vi "BallOutOfFieldRole.vi"(8 "error in (no error)":errorcluster, 10 "Game in":refnum<class "Game.lvclass">, 11 "BallOutOfFieldRole in":refnum<class "BallOutOfFieldRole.lvclass">) -> (0 "error out":errorcluster, 1 "Game out":refnum<class "Game.lvclass">, 2 "Robot out":refnum<class "Robot.lvclass">, 3 "BallOutOfFieldRole out":refnum<class "BallOutOfFieldRole.lvclass">)   [LabVIEW 2018, in "BallOutOfFieldRole.lvclass"]
uses:
  BallOutOfFieldRole.lvclass
  AttackerBallOutOfFieldTactic_class/AttackerBallOutOfFieldTactic.lvclass
  Tacticbook_class/Tacticbook.lvclass
  AttackerBallOutOfFieldTactic_class/States.ctl
  Game_class/Game.lvclass
  Robot_class/Robot.lvclass
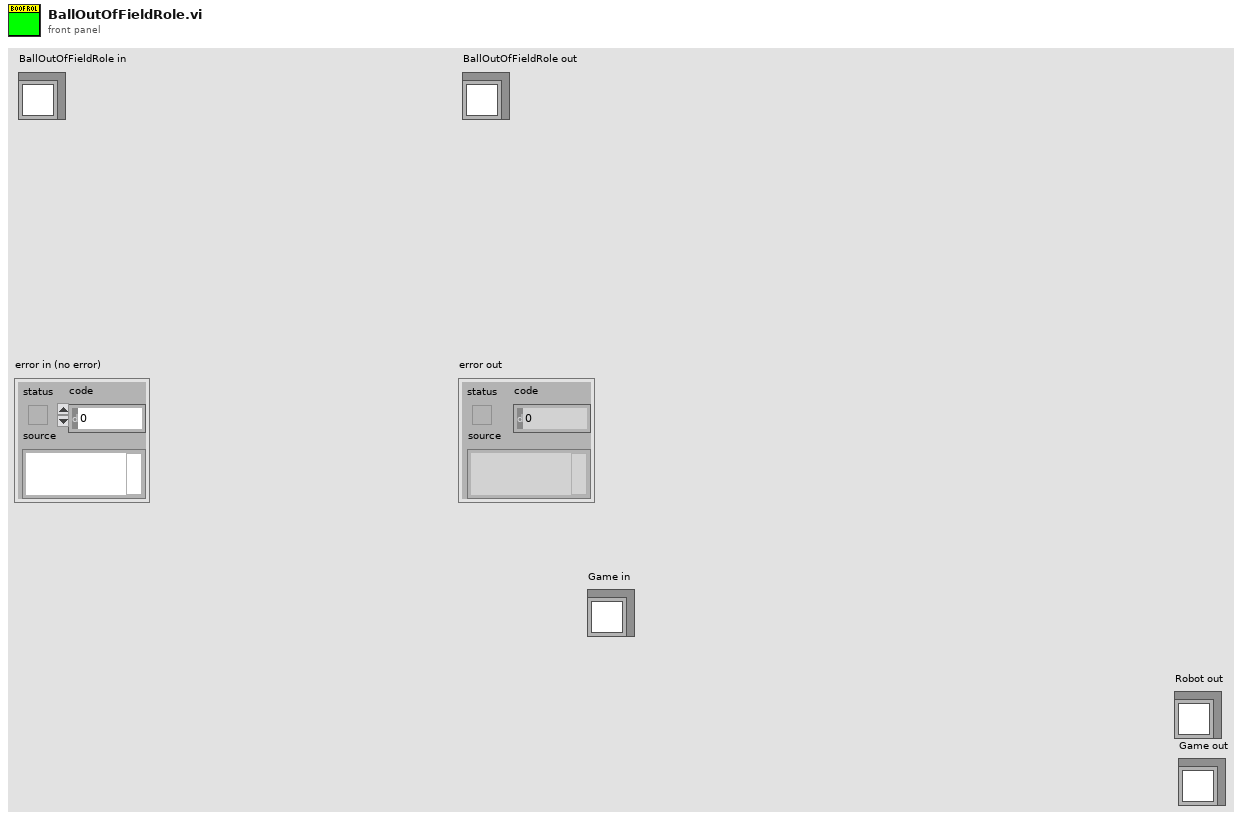
[diagram p1: front panel]
types:
  T1 = typedef "AttackerBallOutOfFieldTactic.lvclass/States.ctl" = enum16{"Exit", "BallOutOfField"}
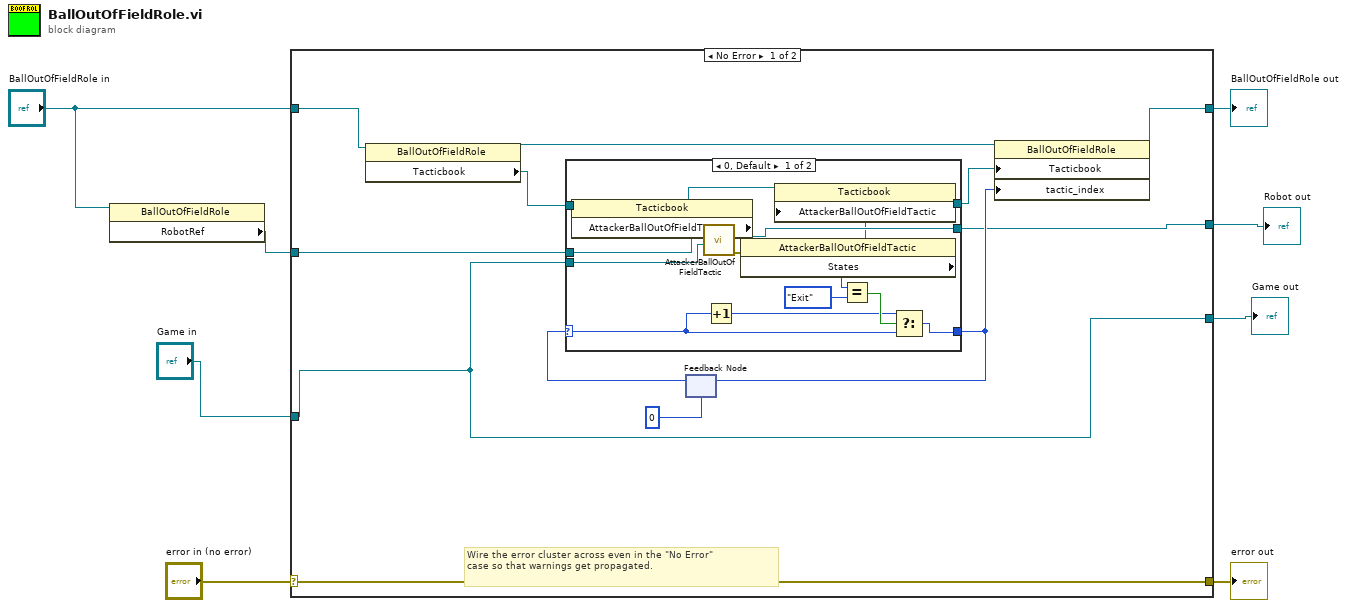
[diagram p0: block diagram]
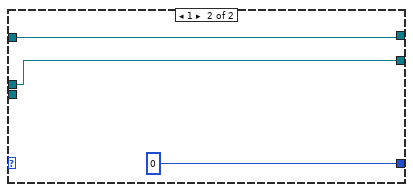
[diagram p2: hidden frame]
diagram:
  n1 = property class="BallOutOfFieldRole"(reference="BallOutOfFieldRole in") -> ("RobotRef"=w5:refnum<class "Robot.lvclass">)  [unwired: 1 in, 2 out]
  n2 = case shown="No Error" "error in (no error)" {
    selector: "error in (no error)" -> [w20 w43]
    tunnel: [w20 w43] -> w7
    tunnel: [w9 w42] -> w6
    tunnel: "BallOutOfFieldRole in" -> [w13 w42]
    tunnel: w5 -> [w12 w41]
    tunnel: "Game in" -> [w11 w40]
    tunnel: [w11 w40] -> w3
    tunnel: [w10 w41] -> w2
    frame No Error {
      # "Wire the error cluster across even in the \"No Error\"\ncase so that warnings get propagated."
      n3 = property class="BallOutOfFieldRole"(reference=w13) -> (reference out=w19:refnum<class "BallOutOfFieldRole.lvclass">, "Tacticbook"=w16:refnum<class "Tacticbook.lvclass">)  [unwired: 1 in, 1 out]
      n4 = feedback #1(0) -> (w17:i32)
      n5 = case shown="0, Default" w17 {
        selector: w17 -> [w27 _]
        tunnel: [w28 0] -> w15
        tunnel: w16 -> [w36 w37]
        tunnel: w12 -> [w34 w39]
        tunnel: [w33 w39] -> w10
        tunnel: [w23 w37] -> w14
        tunnel: w11 -> [w22 _]
        frame 0, Default {
          n6 = property class="Tacticbook"(reference=w36) -> (reference out=w25:refnum<class "Tacticbook.lvclass">, "AttackerBallOutOfFieldTactic"=w35:refnum<class "AttackerBallOutOfFieldTactic.lvclass">)  [unwired: 1 in, 1 out]
          n7 = call-dynamic "AttackerBallOutOfFieldTactic.vi"("Game in"=w22, "Robot"=w34, "AttackerBallOutOfFieldTactic in"=w35) -> ("error out"=w32:errorcluster, "Robot out"=w33:refnum<class "Robot.lvclass">, "AttackerBallOutOfFieldTactic out"=w31:refnum<class "AttackerBallOutOfFieldTactic.lvclass">)  [unwired: 6 in]
          n8 = Increment(x=w27) -> (x+1=w26:i32)
          n9 = property class="AttackerBallOutOfFieldTactic"(reference=w31, error in=w32) -> (reference out=w24:refnum<class "AttackerBallOutOfFieldTactic.lvclass">, "States"=w30:T1)  [unwired: 1 out]
          n10 = property class="Tacticbook"(reference=w25, "AttackerBallOutOfFieldTactic"=w24) -> (reference out=w23:refnum<class "Tacticbook.lvclass">)  [unwired: 1 in, 1 out]
          n11 = Equal?(x=w30, y=States."Exit") -> (x = y?=w29:bool)
          n12 = Select(t=w26, s=w29, f=w27) -> (s? t:f=w28:i32)
        }
        frame 1 {
        }
      }
      n13 = feedback-in #1(w15) -> ()
      n14 = property class="BallOutOfFieldRole"(reference=w19, "Tacticbook"=w14, "tactic_index"=w15) -> (reference out=w9:refnum<class "BallOutOfFieldRole.lvclass">)  [unwired: 1 in, 1 out]
    }
    frame Error {
    }
  }
  "error out" <- w7
  "BallOutOfFieldRole out" <- w6
  "Robot out" <- w2
  "Game out" <- w3
